vi "Status Created Queues.vi"(11 "Base Queue in":refnum<class "Base Queue.lvclass">) -> (0 "Created Queue Count":i32, 1 "Created Queue Aliases":string[](array[string]), 2 "Created Queue Exist?":bool, 3 "Base Queue out":refnum<class "Base Queue.lvclass">)   [LabVIEW 2021, in "jettl.lvlib" / "Base Queue.lvlib" / "Base Queue.lvclass"]
uses:
  Base Queue.lvclass
  C:/git/jettl/src/jettl/jettl/jettl.lvclass
  Base Queue.lvclass/Base Queue.ctl
  Queue Mailbox/Queue Mailbox.lvlib
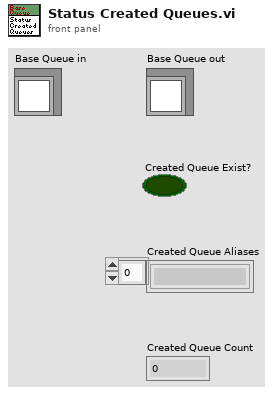
[diagram p1: front panel]
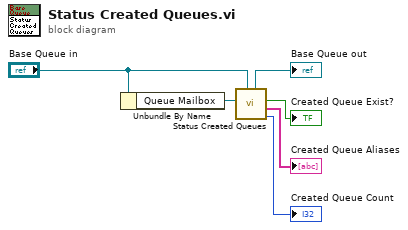
[diagram p0: block diagram]
diagram:
  n1 = Unbundle By Name("Base Queue in") -> ("Queue Mailbox"=w6:refnum<data-value>)
  n2 = call "Status Created Queues.vi"("jettl in"="Base Queue in", "Queue Mailbox"=w6) -> ("Created Queue Count"=→"Created Queue Count":i32, "Created Queue Aliases"=→"Created Queue Aliases":string[], "Created Queue Exist?"=→"Created Queue Exist?":bool, "jettl out"=→"Base Queue out":refnum<class "Base Queue.lvclass">)  [unwired: 6 in]
